vi "Create String.vi"(4 "Heart Rate":u32, 6 "Cadence":dbl, 7 "String in":string, 9 "Power":dbl, 10 "Torque":dbl, 11 "t0":timestamp) -> (3 "String out":string)   [LabVIEW 2013]
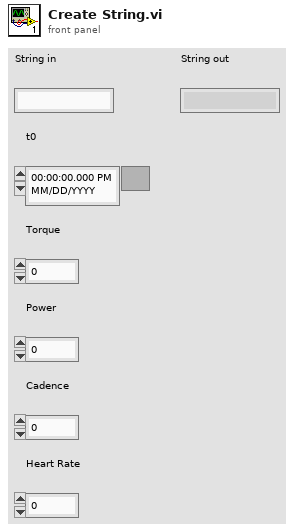
[diagram p1: front panel]
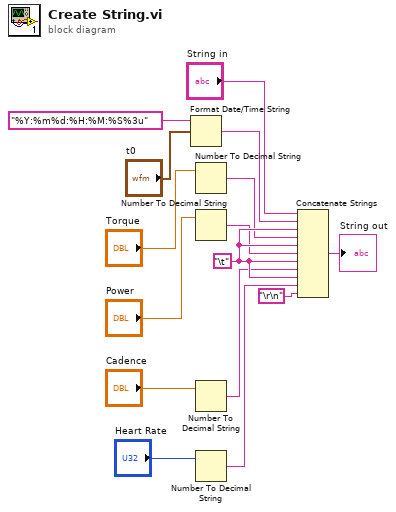
[diagram p0: block diagram]
diagram:
  w13 = "\t"
  n1 = Format Date/Time String(time format string (%c)="%Y:%m%d:%H:%M:%S%3u", seconds (now)="t0") -> (date/time string=w4:string)  [unwired: 1 in]
  n2 = Number To Decimal String(number="Torque") -> (decimal integer string=w7:string)  [unwired: 1 in]
  n3 = Number To Decimal String(number="Power") -> (decimal integer string=w8:string)  [unwired: 1 in]
  n4 = Number To Decimal String(number="Cadence") -> (decimal integer string=w9:string)  [unwired: 1 in]
  n5 = Number To Decimal String(number="Heart Rate") -> (decimal integer string=w14:string)  [unwired: 1 in]
  n6 = Concatenate Strings("String in", w4, w13, w7, w13, w8, w13, w9, w13, w14, "\r\n") -> (→"String out":string)
